vi "Twist2d_GetAll.vi"(11 "TWIST":T1) -> (1 "dTHETA":dbl, 2 "dY":dbl, 3 "dX":dbl)   [LabVIEW 2019, in "Trajectory_Library.lvlib"]
doc: "Get the individual components of the TWIST data structure\n\nParameters:\n - in twist - TWIST data structure\n\nReturns:\n - dx - Linear \"dx\" component.\n - dy - Linear \"dy\" component.\n - dtheta - Angular \"dtheta\" component (radians)."
uses:
  Trajectory_Library.lvlib
  TypeDef/TWIST2D.ctl
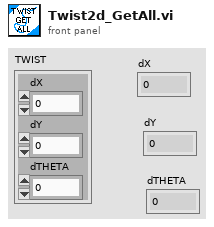
[diagram p1: front panel]
types:
  T1 = typedef "Trajectory_Library.lvlib/TWIST2D.ctl" = cluster{"dX":dbl, "dY":dbl, "dTHETA":dbl}
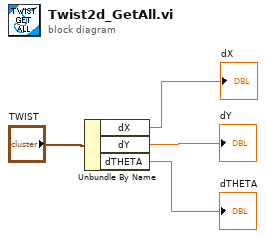
[diagram p0: block diagram]
diagram:
  n1 = Unbundle By Name("TWIST") -> ("dX"=→"dX":dbl, "dY"=→"dY":dbl, "dTHETA"=→"dTHETA":dbl)
